vi "MiliSec to Time string.vi"(11 "mSec interval":u32) -> (2 "Time String":string)   [LabVIEW 2018]
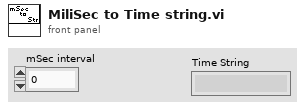
[diagram p1: front panel]
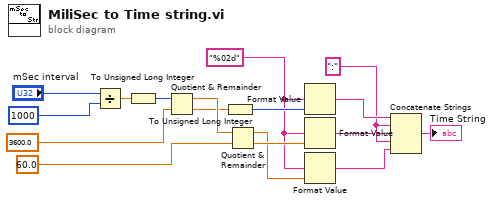
[diagram p0: block diagram]
diagram:
  w2 = "%02d" ("format string")
  w9 = ":" ("string")
  n1 = Divide(x="mSec interval", y=u32 1000 ("x")) -> (x/y=w15:dbl)
  n2 = To Unsigned Long Integer(number=w15) -> (unsigned 32bit integer=w1:u32)
  n3 = Quotient & Remainder(x=w1, y=3600.0 ("value")) -> (x-y*floor(x/y)=w12:dbl, floor(x/y)=w10:dbl)
  n4 = To Unsigned Long Integer(number=w10) -> (unsigned 32bit integer=w7:u32)
  n5 = Quotient & Remainder(x=w12, y=60.0 ("value")) -> (x-y*floor(x/y)=w3:dbl, floor(x/y)=w6:dbl)
  n6 = Format Value(format string=w2, value (0)=w7) -> (output string=w11:string)  [unwired: 1 in]
  n7 = Format Value(format string=w2, value (0)=w6) -> (output string=w5:string)  [unwired: 1 in]
  n8 = Format Value(format string=w2, value (0)=w3) -> (output string=w4:string)  [unwired: 1 in]
  n9 = Concatenate Strings(w11, w9, w5, w9, w4) -> (→"Time String":string)
